vi "Loop Async.vi"(6 "MultiErrors":refnum<class "MultiErrors.lvclass">, 7 "VolatusAPI":refnum<class "VolatusAPI.lvclass">, 8 "Sequencer":refnum<class "MessageQ.lvclass">, 9 "Promise":refnum<class "Promise.lvclass">, 10 "Sequence Config":refnum<class "Sequence Config.lvclass">, 11 "Sequence in":refnum<class "Sequence.lvclass">) -> ()   [LabVIEW 2023, in "VolatusSeq.lvlib" / "Sequence.lvclass"]
uses:
  Sequence.lvclass
  lv-promises/Promises/Promise/Promise.lvclass
  Volatus/VolatusAPI/VolatusAPI.lvclass
  VolatusSeqConfig/Sequence Config/Sequence Config.lvclass
  Volatus/MessageQ/MessageQ.lvclass
  VolatusErrorUtilities/MultiErrors/MultiErrors.lvclass
  lv-promises/Promises/Value/Value.lvclass
  VolatusErrorUtilities/MultiErrors/MultiErrors.lvclass/MultiErrors.ctl
  Sequence.lvclass/Sequence.ctl
  State/State.lvclass
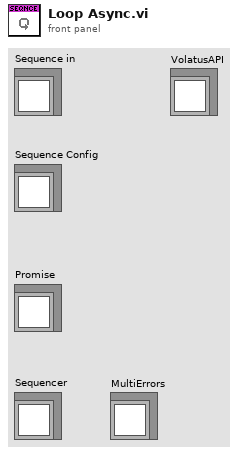
[diagram p1: front panel]
types:
  T1 = typedef "VolatusSeq.lvlib/Sequence.lvclass/Loop Data.ctl" = cluster{"States":map{string, refnum<class "State.lvclass">}, "State":string, "Running":bool, "Seq Start":dbl, "State Start":dbl, "Sequencer":refnum<class "MessageQ.lvclass">, "Time":T2, "Entry State":string, "Abort State":string, "Reset":bool, "Started":dbl, "Last Report":dbl, "Transition":bool, "Debug":T3}
  T2 = typedef "VolatusSeq.lvlib/Sequence Time.ctl" = cluster{"Abort":bool, "Seq Time":dbl, "State Time":dbl, "Wall Time":dbl}
  T3 = typedef "VolatusSeqConfig.lvlib/Debug Flags.ctl" = cluster{"States":bool, "Conditions":bool, "Timing":bool}
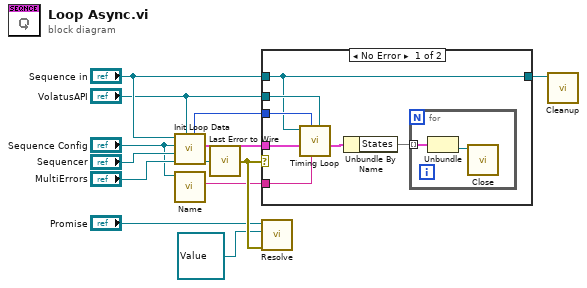
[diagram p0: block diagram]
diagram:
  n1 = call "Init Loop Data.vi"("VolatusAPI"="VolatusAPI", "error in (no error)"="MultiErrors", "Sequencer"="Sequencer", "Sequence Config"="Sequence Config", "Sequence in"="Sequence in") -> ("error out"=w12:refnum<class "MultiErrors.lvclass">, "Loop Data"=w11:T1, "Period"=w3:i64)  [unwired: 3 in, 1 out]
  n2 = call "Name.vi"("Sequence Config in"="Sequence Config") -> ("Name"=w1:string)  [unwired: 8 in, 2 out]
  n3 = call "Last Error to Wire.vi"("MultiErrors in"=w12) -> ("error out"=w13:errorcluster)  [unwired: 8 in]
  n4 = case shown="No Error" w13 {
    tunnel: w11 -> [w19 _]
    tunnel: "Sequence in" -> [w15 w23]
    tunnel: "VolatusAPI" -> [w16 _]
    tunnel: [w15 w23] -> w7
    tunnel: w3 -> [w17 _]
    tunnel: w1 -> [w14 _]
    frame No Error {
      n5 = call "Timing Loop.vi"("VolatusAPI"=w16, "Seq Name"=w14, "Period"=w17, "Loop Data in"=w19, "Sequence in"=w15) -> ("Loop Data"=w18:T1)  [unwired: 6 in]
      n6 = Unbundle By Name(w18) -> ("States"=w20:map{string, refnum<class "State.lvclass">})
      n7 = for {
        tunnel: w20 -> [w22] mode=indexing
        n8 = Unbundle(w22) -> ("State"=w21:refnum<class "State.lvclass">)  [unwired: 1 out]
        n9 = call "Close.vi"("State in"=w21) -> ()  [unwired: 10 in, 1 out]
      }
    }
    frame Error {
    }
  }
  n10 = call "Resolve.vi"("error in (no error)"=w13, "Result (None)"=refnum<class "Value.lvclass"> refnum ("Result"), "Promise in"="Promise") -> ()  [unwired: 7 in, 2 out]
  n11 = call "Cleanup.vi"("Sequence in"=w7) -> ()  [unwired: 10 in, 1 out]
